vi "write_DAC_word.vi"(7 "converter box version":i16=1 min=1 max=2, 10 "U16 data number":u16, 11 "DAC values in":T1 {"bit index" min=-1 max=17 step=1; "channel index" max=7 step=1; "offset" max=4095; "DAC voltage"."ch1" max=4095 step=1; "DAC voltage"."ch0" max=4095 step=1}) -> (3 "DAC values out":T1 {"bit index" min=-1 max=17 step=1; "channel index" max=7 step=1; "offset" max=4095; "DAC voltage"."ch1" max=4095 step=1; "DAC voltage"."ch0" max=4095 step=1})   [LabVIEW 2010]
uses:
  FPGA_Typedefs/DAC_values_cluster.ctl
  FPGA_Typedefs/DAC_voltage_cluster.ctl
  <vilib>/eio/EIONode/EIONode.xnode
  <vilib>/rvi/eio/nirviEIOImplementation/nirviEIOImplementation.xnode
  <vilib>/rvi/eio/common/nirviEmuClasses.ctl
  <vilib>/rvi/eio/common/nirviEmuTemplateMethod_noerrors.vi
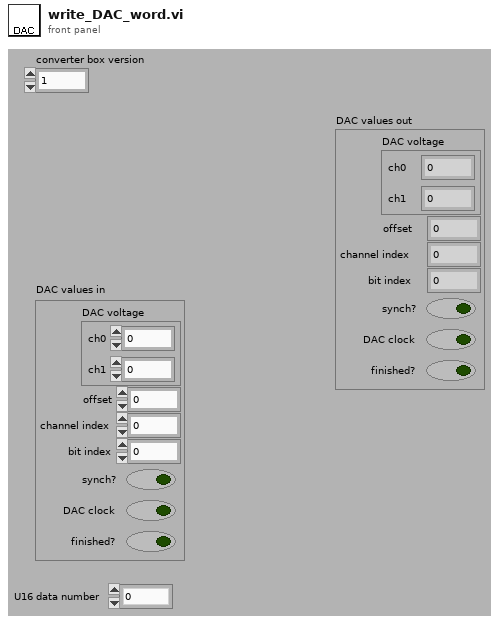
[diagram p1: front panel]
types:
  T1 = typedef "DAC_values_cluster.ctl" = cluster{"DAC voltage":T2, "offset":u16, "channel index":u16, "bit index":i32, "synch?":bool, "DAC clock":bool, "finished?":bool}
  T2 = typedef "DAC_voltage_cluster.ctl" = cluster{"ch0":u16, "ch1":u16}
  T3 = typedef "nirviEmuClasses.ctl" = enum16{"IO Read", "IO Write", "Method", "Property Read", "Property Write"}
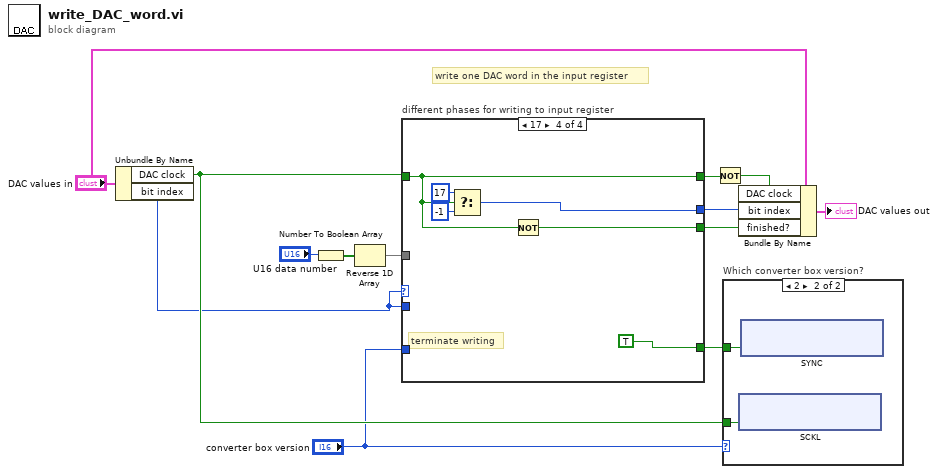
[diagram p0: block diagram]
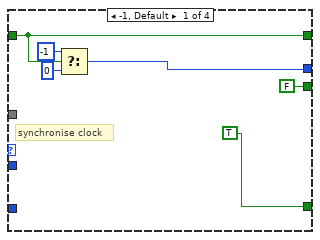
[diagram p3: hidden frame]
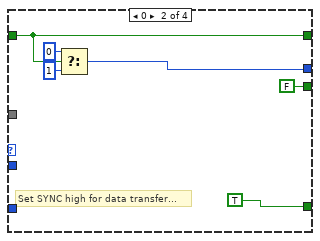
[diagram p4: hidden frame]
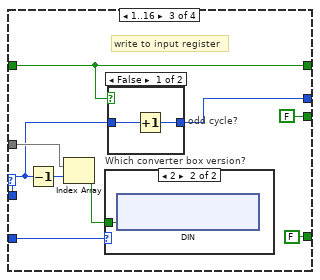
[diagram p5: hidden frame]
diagram:
  # "write one DAC word in the input register"
  n1 = Unbundle By Name("DAC values in") -> ("DAC clock"=w8:bool, "bit index"=w7:i32)
  n2 = Number To Boolean Array(number="U16 data number") -> (Boolean array=w13:bool[])
  n3 = Reverse 1D Array(array=w13) -> (reversed array=w11:bool[])
  n4 = case "different phases for writing to input register" shown="17" w7 {
    tunnel: w8 -> [w17 w21 w32 w51]
    tunnel: [w16 w23 w30 w53] -> w4
    tunnel: [TRUE ("SYNC") TRUE ("SYNC") FALSE ("SYNC") TRUE ("SYNC")] -> w9
    tunnel: w7 -> [_ _ w31 _]
    tunnel: w11 -> [_ _ w33 _]
    tunnel: [w17 w21 w32 w51] -> w10
    tunnel: [FALSE FALSE FALSE w50] -> w3
    tunnel: "converter box version" -> [_ _ w27 _]
    frame -1, Default {
      # "synchronise clock"
      n5 = Select(t=-1, s=w17, f=0) -> (s? t:f=w16:i32)
    }
    frame 0 {
      # "Set SYNC high for data transfer..."
      n6 = Select(t=0, s=w21, f=1) -> (s? t:f=w23:i32)
    }
    frame 1..16 {
      # "write to input register"
      n7 = Decrement(x=w31) -> (x-1=w34:i32)
      n8 = Index Array(array=w33, index=w34) -> (element=w28:bool)
      n9 = case "Which converter box version?" shown="2" w27 {
        tunnel: w28 -> [_ w35]
        frame Default {
        }
        frame 2 {
          n10 = xnode "DIN"("Connector1/DIO36"=w35) -> ()  [unwired: 1 in, 1 out]
        }
      }
      n11 = case "odd cycle?" shown="False" w32 {
        tunnel: w31 -> [w47 w49]
        tunnel: [w48 w49] -> w30
        frame False {
          n12 = Increment(x=w47) -> (x+1=w48:i32)
        }
        frame True {
        }
      }
    }
    frame 17 {
      # "terminate writing"
      n13 = Select(t=17, s=w51, f=-1) -> (s? t:f=w53:i32)
      n14 = Not(x=w51) -> (.not. x?=w50:bool)
    }
  }
  n15 = Not(x=w10) -> (.not. x?=w5:bool)
  n16 = case "Which converter box version?" shown="2" "converter box version" {
    tunnel: w9 -> [_ w57]
    tunnel: w8 -> [_ w56]
    frame Default {
    }
    frame 2 {
      n17 = xnode "SCKL"("Connector1/DIO38"=w56) -> ()  [unwired: 1 in, 1 out]
      n18 = xnode "SYNC"("Connector1/DIO34"=w57) -> ()  [unwired: 1 in, 1 out]
    }
  }
  n19 = Bundle By Name(cluster="DAC values in", "DAC clock"=w5, "bit index"=w4, "finished?"=w3) -> (→"DAC values out":T1)
